vi "fgv_load_save.vi"(8 "Error in":errorcluster, 9 "write":bool, 11 "filename_set":string) -> (0 "error out":errorcluster, 3 "filename_get":string)   [LabVIEW 2025]
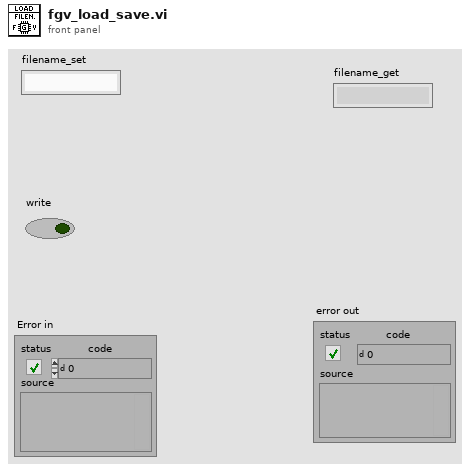
[diagram p1: front panel]
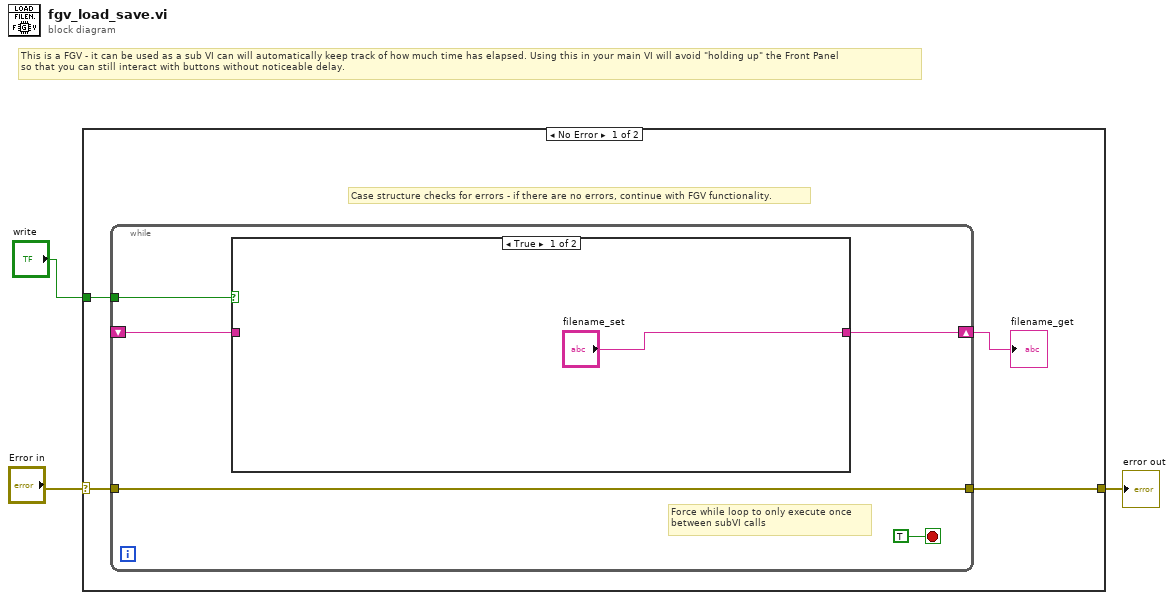
[diagram p0: block diagram]
diagram:
  # "This is a FGV - it can be used as a sub VI can will automatically keep track of how much time has elapsed. Using this in your main VI will avoid \"holding up\" the Front Panel \nso that you can still interact with buttons without noticeable delay."
  n1 = case shown="No Error" "Error in" {
    selector: "Error in" -> [w7 w15]
    tunnel: [w6 w15] -> w2
    tunnel: "write" -> [w5 _]
    frame No Error {
      # "Case structure checks for errors - if there are no errors, continue with FGV functionality."
      n2 = while {
        shift-right: [w10] -> w4
        shift-left: _ -> [w11]
        tunnel: w7 -> [w9]
        tunnel: [w9] -> w6
        tunnel: w5 -> [w8]
        stop <- TRUE stop-if-true
        # "Force while loop to only execute once\nbetween subVI calls"
        n3 = case shown="True" w8 {
          tunnel: w11 -> [_ w14]
          tunnel: ["filename_set" w14] -> w10
          frame True {
          }
          frame False {
          }
        }
      }
      "filename_get" <- w4
    }
    frame Error {
      # "Case structure checks for errors - if there's an errorr, do nothing except pass the error back out"
    }
  }
  "error out" <- w2
